vi "FWHMCalculate.vi"(0 "Lambda":dbl[](array[numeric]), 1 "Spectra":dbl[](array[numeric])) -> (2 "Spectral Results":T1, 3 "Right Band":cluster{dbl[], dbl[]}, 4 "Left Band":cluster{dbl[], dbl[]})   [LabVIEW 2012]
panel:
  out "FWHM Raw":dbl
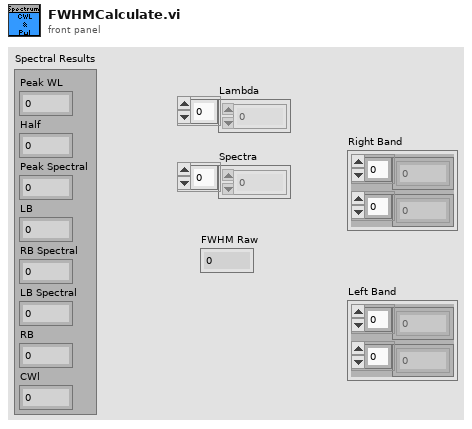
[diagram p1: front panel]
types:
  T1 = cluster{"Peak WL":dbl, "Half":dbl, "Peak Spectral":dbl, "LB":dbl, "RB Spectral":dbl, "LB Spectral":dbl, "RB":dbl, "CWl":dbl}
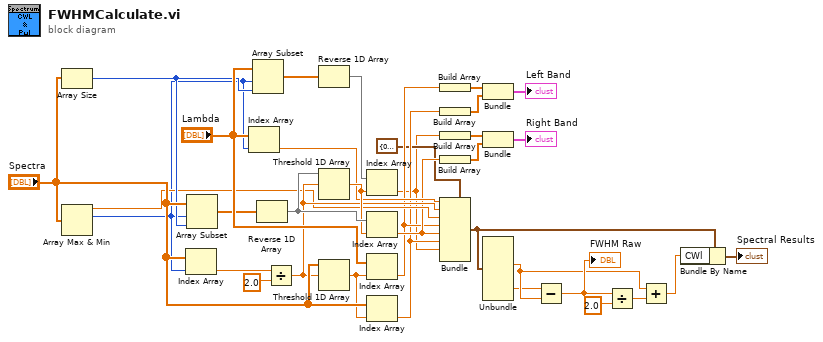
[diagram p0: block diagram]
diagram:
  n1 = Array Size(array="Spectra") -> (size(s)=w26:i32)
  n2 = Array Max & Min(array="Spectra") -> (max value=w16:dbl, max index (indices)=w15:i32)  [unwired: 2 out]
  n3 = Index Array(array="Spectra", index=w15) -> (element=w25:dbl)
  n4 = Array Subset(array="Spectra", index=w15, length=w26) -> (w27:dbl[])
  n5 = Index Array "Index Array"(array="Lambda", index=w15) -> (element=w14:dbl)
  n6 = Array Subset(array="Lambda", index=w15, length=w26) -> (w28:dbl[])
  n7 = Reverse 1D Array(array=w27) -> (reversed array=w31:dbl[])
  n8 = Divide(x=w25, y=2.0) -> (x/y=w17:dbl)
  n9 = Reverse 1D Array(array=w28) -> (reversed array=w29:dbl[])
  n10 = Threshold 1D Array(2:w17, 3:w31) -> (0:w30:dbl)  [unwired: 1 in]
  n11 = Threshold 1D Array(2:w17, 3:"Spectra") -> (0:w32:dbl)  [unwired: 1 in]
  n12 = Index Array(array=w29, index=w30) -> (element=w9:dbl)
  n13 = Index Array(array=w31, index=w30) -> (element=w13:dbl)
  n14 = Index Array(array="Lambda", index=w32) -> (element=w12:dbl)
  n15 = Index Array(array="Spectra", index=w32) -> (element=w11:dbl)
  n16 = Build Array(w12) -> (w20:dbl[])
  n17 = Build Array(w11) -> (w19:dbl[])
  n18 = Build Array(w9) -> (w23:dbl[])
  n19 = Build Array(w13) -> (w22:dbl[])
  n20 = Bundle(cluster=T1 {"Peak WL"=0.0, "Half"=0.0, "Peak Spectral"=0.0, "LB"=0.0, "RB Spectral"=0.0, "LB Spectral"=0.0, "RB"=0.0, "CWl"=0.0} ("Spectral Results"), "Peak WL"=w14, "Half"=w17, "Peak Spectral"=w16, "LB"=w12, "RB Spectral"=w13, "LB Spectral"=w11, "RB"=w9) -> (w3:T1)  [unwired: 1 in]
  n21 = Bundle(w20, w19) -> (→"Left Band":cluster{dbl[], dbl[]})  [unwired: 1 in]
  n22 = Bundle(w23, w22) -> (→"Right Band":cluster{dbl[], dbl[]})  [unwired: 1 in]
  n23 = Unbundle(w3) -> ("LB"=w5:dbl, "RB"=w4:dbl)  [unwired: 6 out]
  n24 = Subtract(x=w4, y=w5) -> (x-y=w8:dbl)
  "FWHM Raw" <- w8
  n25 = Divide(x=w8, y=2.0) -> (x/y=w6:dbl)
  n26 = Add(x=w5, y=w6) -> (x+y=w2:dbl)
  n27 = Bundle By Name(cluster=w3, "CWl"=w2) -> (→"Spectral Results":T1)
